vi "load_select.vi"(8 "error in":errorcluster) -> (0 "error out":errorcluster, 3 "Array":string[](array[string]))   [LabVIEW 2012]
panel:
  in  "Microwave":bool
  in  "Switches":bool
  in  "Frequency":bool
  in  "Time":bool
  in  "OK":bool
  in  "Data":bool
  in  "Waveplates":bool
  in  "Wavemaster":bool
  in  "Commands":bool
  in  "DDG":bool
  in  "Trap DDS":bool
  in  "AOM DDS":bool
  in  "Lasers":bool
  in  "Scan":bool
  in  "DAC":bool
  in  "DIO64":bool
  in  "Everything":bool
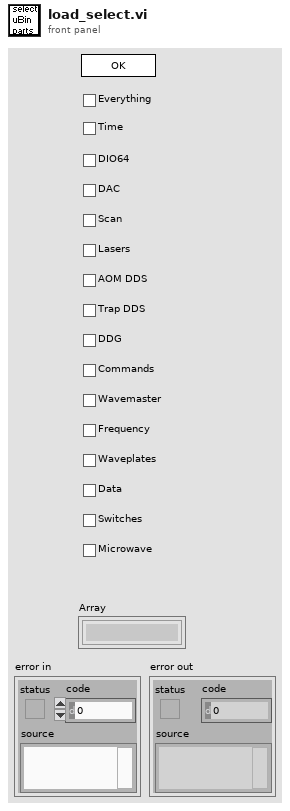
[diagram p1: front panel]
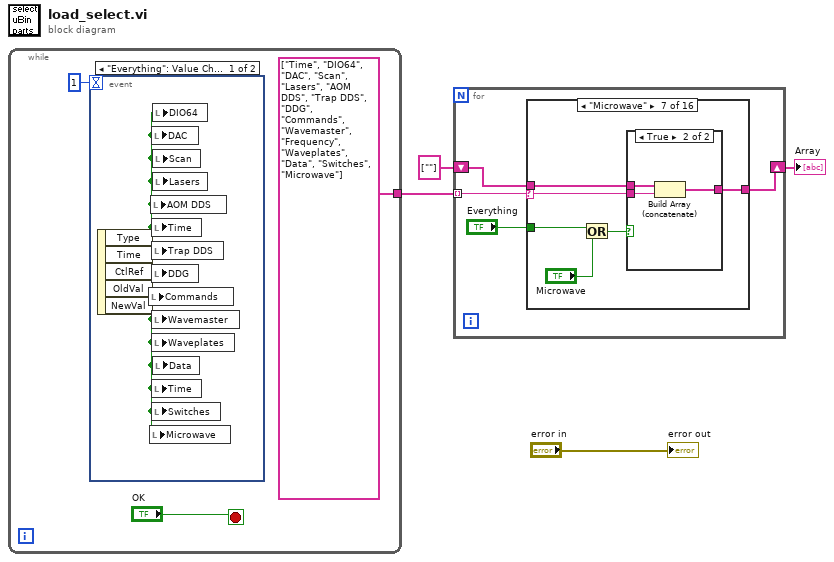
[diagram p0: block diagram]
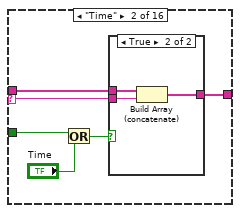
[diagram p3: hidden frame]
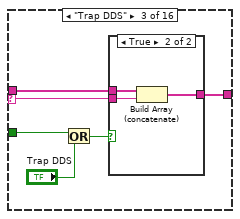
[diagram p5: hidden frame]
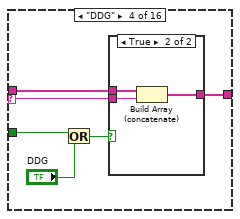
[diagram p7: hidden frame]
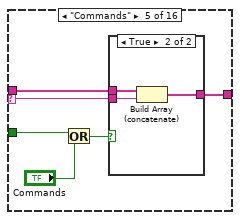
[diagram p9: hidden frame]
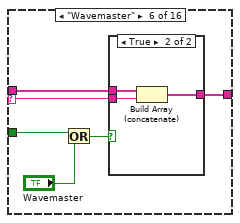
[diagram p11: hidden frame]
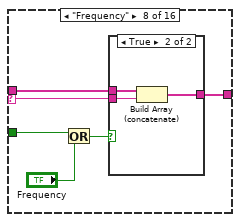
[diagram p14: hidden frame]
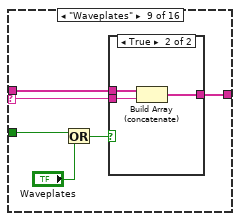
[diagram p16: hidden frame]
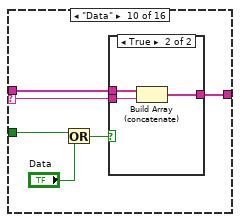
[diagram p18: hidden frame]
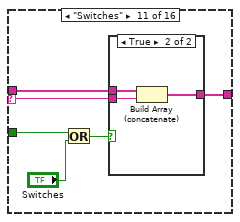
[diagram p20: hidden frame]
diagram:
  n1 = while {
    tunnel: [string[] ["Time", "DIO64", "DAC", "Scan", "Lasers", "AOM DDS", "Trap DDS", "DDG", "Commands", "Wavemaster", "Frequency", "Waveplates", "Data", "Switches", "Microwave"]] -> w4
    stop <- "OK" stop-if-true
    n2 = event shown="[0] \"Everything\": Value Change" {
      selector: _ -> [_ _]
      dyn-events: _ -> [_ _]
      timeout: 1 -> [_ _]
      event "Everything": Value Change {
        n3 = event-data() -> ("NewVal"=w8:bool)  [unwired: 1 in, 4 out]
        n4 = local write "Commands"(w8) -> ()
        n5 = local write "Microwave"(w8) -> ()
        n6 = local write "AOM DDS"(w8) -> ()
        n7 = local write "DAC"(w8) -> ()
        n8 = local write "Time"(w8) -> ()
        n9 = local write "Trap DDS"(w8) -> ()
        n10 = local write "DDG"(w8) -> ()
        n11 = local write "Wavemaster"(w8) -> ()
        n12 = local write "Waveplates"(w8) -> ()
        n13 = local write "Time"(w8) -> ()
        n14 = local write "Switches"(w8) -> ()
        n15 = local write "DIO64"(w8) -> ()
        n16 = local write "Scan"(w8) -> ()
        n17 = local write "Lasers"(w8) -> ()
        n18 = local write "Data"(w8) -> ()
      }
      event Timeout {
        n19 = event-data() -> ()  [unwired: 1 in, 3 out]
      }
    }
  }
  n20 = for {
    tunnel: w4 -> [w12] mode=indexing
    shift-right: [w9] -> w2
    shift-left: string[] [""] -> [w10]
    n21 = case shown="\"Microwave\"" w12 {
      selector: w12 -> [_ w16 w27 w37 w47 w57 w67 w77 w87 w97 w107 w118 w128 w138 w148 w158]
      tunnel: "Everything" -> [_ w19 w29 w39 w49 w59 w69 w79 w89 w99 w109 w119 w129 w139 w149 w159]
      tunnel: w10 -> [w13 w15 w26 w36 w46 w56 w66 w76 w86 w96 w106 w117 w127 w137 w147 w157]
      tunnel: [w13 w14 w25 w35 w45 w55 w65 w75 w85 w95 w105 w116 w126 w136 w146 w156] -> w9
      frame "False", Default {
      }
      frame "Time" {
        n22 = Or(x=w19, y="Time") -> (x .or. y?=w17:bool)
        n23 = case shown="True" w17 {
          tunnel: w16 -> [_ w23]
          tunnel: w15 -> [w20 w22]
          tunnel: [w20 w21] -> w14
          frame False {
          }
          frame True {
            n24 = Build Array (concatenate)(w22, w23) -> (w21:string[])
          }
        }
      }
      frame "Trap DDS" {
        n25 = Or(x=w29, y="Trap DDS") -> (x .or. y?=w28:bool)
        n26 = case shown="True" w28 {
          tunnel: w27 -> [_ w33]
          tunnel: w26 -> [w30 w32]
          tunnel: [w30 w31] -> w25
          frame False {
          }
          frame True {
            n27 = Build Array (concatenate)(w32, w33) -> (w31:string[])
          }
        }
      }
      frame "DDG" {
        n28 = Or(x=w39, y="DDG") -> (x .or. y?=w38:bool)
        n29 = case shown="True" w38 {
          tunnel: w37 -> [_ w43]
          tunnel: w36 -> [w40 w42]
          tunnel: [w40 w41] -> w35
          frame False {
          }
          frame True {
            n30 = Build Array (concatenate)(w42, w43) -> (w41:string[])
          }
        }
      }
      frame "Commands" {
        n31 = Or(x=w49, y="Commands") -> (x .or. y?=w48:bool)
        n32 = case shown="True" w48 {
          tunnel: w47 -> [_ w53]
          tunnel: w46 -> [w50 w52]
          tunnel: [w50 w51] -> w45
          frame False {
          }
          frame True {
            n33 = Build Array (concatenate)(w52, w53) -> (w51:string[])
          }
        }
      }
      frame "Wavemaster" {
        n34 = Or(x=w59, y="Wavemaster") -> (x .or. y?=w58:bool)
        n35 = case shown="True" w58 {
          tunnel: w57 -> [_ w63]
          tunnel: w56 -> [w60 w62]
          tunnel: [w60 w61] -> w55
          frame False {
          }
          frame True {
            n36 = Build Array (concatenate)(w62, w63) -> (w61:string[])
          }
        }
      }
      frame "Microwave" {
        n37 = Or(x=w69, y="Microwave") -> (x .or. y?=w68:bool)
        n38 = case shown="True" w68 {
          tunnel: w67 -> [_ w73]
          tunnel: w66 -> [w70 w72]
          tunnel: [w70 w71] -> w65
          frame False {
          }
          frame True {
            n39 = Build Array (concatenate)(w72, w73) -> (w71:string[])
          }
        }
      }
      frame "Frequency" {
        n40 = Or(x=w79, y="Frequency") -> (x .or. y?=w78:bool)
        n41 = case shown="True" w78 {
          tunnel: w77 -> [_ w83]
          tunnel: w76 -> [w80 w82]
          tunnel: [w80 w81] -> w75
          frame False {
          }
          frame True {
            n42 = Build Array (concatenate)(w82, w83) -> (w81:string[])
          }
        }
      }
      frame "Waveplates" {
        n43 = Or(x=w89, y="Waveplates") -> (x .or. y?=w88:bool)
        n44 = case shown="True" w88 {
          tunnel: w87 -> [_ w93]
          tunnel: w86 -> [w90 w92]
          tunnel: [w90 w91] -> w85
          frame False {
          }
          frame True {
            n45 = Build Array (concatenate)(w92, w93) -> (w91:string[])
          }
        }
      }
      frame "Data" {
        n46 = Or(x=w99, y="Data") -> (x .or. y?=w98:bool)
        n47 = case shown="True" w98 {
          tunnel: w97 -> [_ w103]
          tunnel: w96 -> [w100 w102]
          tunnel: [w100 w101] -> w95
          frame False {
          }
          frame True {
            n48 = Build Array (concatenate)(w102, w103) -> (w101:string[])
          }
        }
      }
      frame "Switches" {
        n49 = Or(x=w109, y="Switches") -> (x .or. y?=w108:bool)
        n50 = case shown="True" w108 {
          tunnel: w107 -> [_ w113]
          tunnel: w106 -> [w110 w112]
          tunnel: [w110 w111] -> w105
          frame False {
          }
          frame True {
            n51 = Build Array (concatenate)(w112, w113) -> (w111:string[])
          }
        }
      }
      frame "DIO64" {
        n52 = Or(x=w119, y="DIO64") -> (x .or. y?=w115:bool)
        n53 = case shown="True" w115 {
          tunnel: w118 -> [_ w123]
          tunnel: w117 -> [w120 w122]
          tunnel: [w120 w121] -> w116
          frame False {
          }
          frame True {
            n54 = Build Array (concatenate)(w122, w123) -> (w121:string[])
          }
        }
      }
      frame "DAC" {
        n55 = Or(x=w129, y="DAC") -> (x .or. y?=w125:bool)
        n56 = case shown="True" w125 {
          tunnel: w128 -> [_ w133]
          tunnel: w127 -> [w130 w132]
          tunnel: [w130 w131] -> w126
          frame False {
          }
          frame True {
            n57 = Build Array (concatenate)(w132, w133) -> (w131:string[])
          }
        }
      }
      frame "Scan" {
        n58 = Or(x=w139, y="Scan") -> (x .or. y?=w135:bool)
        n59 = case shown="True" w135 {
          tunnel: w138 -> [_ w143]
          tunnel: w137 -> [w140 w142]
          tunnel: [w140 w141] -> w136
          frame False {
          }
          frame True {
            n60 = Build Array (concatenate)(w142, w143) -> (w141:string[])
          }
        }
      }
      frame "Lasers" {
        n61 = Or(x=w149, y="Lasers") -> (x .or. y?=w145:bool)
        n62 = case shown="True" w145 {
          tunnel: w148 -> [_ w153]
          tunnel: w147 -> [w150 w152]
          tunnel: [w150 w151] -> w146
          frame False {
          }
          frame True {
            n63 = Build Array (concatenate)(w152, w153) -> (w151:string[])
          }
        }
      }
      frame "AOM DDS" {
        n64 = Or(x=w159, y="AOM DDS") -> (x .or. y?=w155:bool)
        n65 = case shown="True" w155 {
          tunnel: w158 -> [_ w163]
          tunnel: w157 -> [w160 w162]
          tunnel: [w160 w161] -> w156
          frame False {
          }
          frame True {
            n66 = Build Array (concatenate)(w162, w163) -> (w161:string[])
          }
        }
      }
    }
  }
  "Array" <- w2
  "error out" <- "error in"
